vi "Modules global.vi"() -> ()   [LabVIEW 2017]
panel:
  out "Error message":string="Done."
  in  "Use backup file":bool
  in  "Read/Write":bool
  in  "Do Write/Read":bool
  in  "filename":string="24_Apr_2007"
  in  "DAC Break":bool
  in  "DAC Loop":bool
  in  "DAC Update":bool
  in  "All Info":T1(array[cluster])=[[{"Port"=0, "Line"=0, "Description"="Scope Trigger", "Default"=FALSE}, {"Port"=0, "Line"=1, "Description"="Camera trigger (On=High)", "Default"=FALSE}, {"Port"=0, "Line"=2, "Description"="Shim (F/B, U/D) Relay (On = High)", "Default"=TRUE}, {"Port"=0, "Line"=3, "Description"="Shim (L/R) Relay (On = High)", "Default"=TRUE}, {"Port"=0, "Line"=4, "Description"="Rb Trap shutter (High = On)", "Default"=TRUE}, {"Port"=0, "Line"=5, "Description"="", "Default"=FALSE}, {"Port"=0, "Line"=6, "Description"="**//bad TTL//", "Default"=FALSE}, {"Port"=0, "Line"=7, "Description"="Rb F=2 probe shutter", "Default"=FALSE}, {"Port"=0, "Line"=8, "Description"="Rb repump shutter", "Default"=TRUE}, {"Port"=0, "Line"=9, "Description"="Na trap Shutter (On=high)", "Default"=TRUE}, {"Port"=0, "Line"=10, "Description"="Na repump shutter(on)", "Default"=TRUE}, {"Port"=0, "Line"=11, "Description"="optical trap on/off", "Default"=FALSE}, {"Port"=0, "Line"=12, "Description"="Na repump VCO TTL", "Default"=TRUE}, {"Port"=0, "Line"=13, "Description"="Na repump II shtter", "Default"=FALSE}, {"Port"=0, "Line"=14, "Description"="Na trap VCO TTL", "Default"=TRUE}, {"Port"=0, "Line"=15, "Description"="Na F = 2 probe VCO TTL", "Default"=FALSE}], [{"Port"=1, "Line"=0, "Description"="UV LED (On=High)", "Default"=FALSE}, {"Port"=1, "Line"=1, "Description"="Rb F = 2 probe VCO TTL", "Default"=FALSE}, {"Port"=1, "Line"=2, "Description"="", "Default"=FALSE}, {"Port"=1, "Line"=3, "Description"="Track Trigger (Low=MOT)", "Default"=FALSE}, {"Port"=1, "Line"=4, "Description"="Quad enable (High=enabled)", "Default"=FALSE}, {"Port"=1, "Line"=5, "Description"="Bias Multiplexer enable (High=enabled)", "Default"=FALSE}, {"Port"=1, "Line"=6, "Description"="**//bad TTL//", "Default"=FALSE}, {"Port"=1, "Line"=7, "Description"="Rb Repump AOM", "Default"=TRUE}, {"Port"=1, "Line"=8, "Description"="shutter for blocking probe direction", "Default"=FALSE}, {"Port"=1, "Line"=9, "Description"="OP magnetic coil", "Default"=FALSE}, {"Port"=1, "Line"=10, "Description"="\"1\" control bit  for Bias servo mux", "Default"=FALSE}, {"Port"=1, "Line"=11, "Description"="\"2\" control bit  for Bias servo mux", "Default"=FALSE}, {"Port"=1, "Line"=12, "Description"="triggering Agilent frequency sweep for ARPing", "Default"=FALSE}, {"Port"=1, "Line"=13, "Description"="triggering Agilent ramp for frequency sweep", "Default"=FALSE}, {"Port"=1, "Line"=14, "Description"="Na probe shutter", "Default"=FALSE}, {"Port"=1, "Line"=15, "Description"="RF switch for Evap of Rb", "Default"=FALSE}], [{"Port"=2, "Line"=0, "Description"="Feshbach coil switch enable", "Default"=FALSE}, {"Port"=2, "Line"=1, "Description"="Feshbach coil switch polarity", "Default"=FALSE}, {"Port"=2, "Line"=2, "Description"="< line unused>", "Default"=FALSE}, {"Port"=2, "Line"=3, "Description"="690 nm Raman Laser shutter", "Default"=FALSE}, {"Port"=2, "Line"=4, "Description"="< line unused>", "Default"=FALSE}, {"Port"=2, "Line"=5, "Description"="< line unused>", "Default"=FALSE}, {"Port"=2, "Line"=6, "Description"="**//bad TTL//", "Default"=FALSE}, {"Port"=2, "Line"=7, "Description"="< line unused>", "Default"=FALSE}, {"Port"=2, "Line"=8, "Description"="E-field plate switch", "Default"=FALSE}, {"Port"=2, "Line"=9, "Description"=" Ti:sapphire (Raman) shutter", "Default"=FALSE}, {"Port"=2, "Line"=10, "Description"="Raman lasers AOM", "Default"=FALSE}, {"Port"=2, "Line"=11, "Description"="STIRAP waveform trigger", "Default"=FALSE}, {"Port"=2, "Line"=12, "Description"="magic box  RF switch", "Default"=FALSE}, {"Port"=2, "Line"=13, "Description"="Na blast AOM", "Default"=FALSE}, {"Port"=2, "Line"=14, "Description"="< line unused >", "Default"=FALSE}, {"Port"=2, "Line"=15, "Description"="new camera trigger (still connected?)", "Default"=FALSE}], [{"Port"=3, "Line"=0, "Description"="IPG AOM trigger", "Default"=FALSE}, {"Port"=3, "Line"=1, "Description"="660 nm laser (probe) AOM", "Default"=FALSE}, {"Port"=3, "Line"=2, "Description"="< line unused>", "Default"=FALSE}, {"Port"=3, "Line"=3, "Description"="< line unused >", "Default"=FALSE}, {"Port"=3, "Line"=4, "Description"="Pinch servo multiplexer enable", "Default"=FALSE}, {"Port"=3, "Line"=5, "Description"="< line unused >", "Default"=FALSE}, {"Port"=3, "Line"=6, "Description"="**//bad TTL//", "Default"=FALSE}, {"Port"=3, "Line"=7, "Description"="< line unused >", "Default"=FALSE}, {"Port"=3, "Line"=8, "Description"="enable STIRAP back Raman AOM freq shift", "Default"=FALSE}, {"Port"=3, "Line"=9, "Description"="< line unused>", "Default"=FALSE}, {"Port"=3, "Line"=10, "Description"="< line unused>", "Default"=FALSE}, {"Port"=3, "Line"=11, "Description"="< line unused >", "Default"=FALSE}, {"Port"=3, "Line"=12, "Description"="< line unused >", "Default"=FALSE}, {"Port"=3, "Line"=13, "Description"="Dynamic DAC Trigger", "Default"=FALSE}, {"Port"=3, "Line"=14, "Description"="Board 1 Clock Trigger", "Default"=FALSE}, {"Port"=3, "Line"=15, "Description"="Board 2 Clock Trigger", "Default"=FALSE}]]
  in  "File names":string[](array[string])=["MOT recapture", "Most recent expt", "Quadrupole trap", "MOT fill", "BEC", "FORT with transfers", "ZP beam align", "Test1", "Test2", "Align probe beam", "Test3", "Test4", "Test5", "Blank", "Roundtrip MOT recapture", "IP trap load recapture"]
  in  "Modules":string[](array[string])=["Atom removal 1", "Atom removal 2", "B-field off", "CMOT", "Defaults", "Final B-field ramps", "Fluorescence pulse", "High field", "High field ARP", "Loading cart QT", "Loading sci QT", "Low field", "Low field ARP", "Mol OD image", "Mol picture", "Mol probe pulse", "Molasses", "MOT off", "MOT on", "OD image", "Optical pumping", "OT B-field off", "Picture", "Probe pulse", "QT off for OT", "Quadrupole trap off", "Quadrupole trap", "Quantization axis", "S-G separation", "STIRAP back for imaging", "STIRAP", "TTL high", "TTL low", "GPIB", "Utility Module 1", "Utility Module 2", "Utility Module 3", "Utility Module 4", "Utility Module 5", "Utility Module 6", "Utility Module 7", "Utility Module 8", "Utility Module 9"]
  # "0\n\n1\n\n2\n\n3\n\n4\n\n5\n\n6\n\n7\n\n8\n\n9\n\n10\n\n11\n\n12\n\n13\n\n14\n\n15\n\n16\n\n17\n\n18\n\n19\n\n20\n\n21\n\n22\n\n23\n\n24\n\n25\n\n26\n\n27\n\n28\n\n29\n\n30\n\n31\n\n32\n\n33\n\n34\n\n35\n\n36\n\n37\n\n38\n\n39\n\n40\n\n41\n\n42\n\n43\n\n44\n\n45\n\n46\n\n47\n\n48"
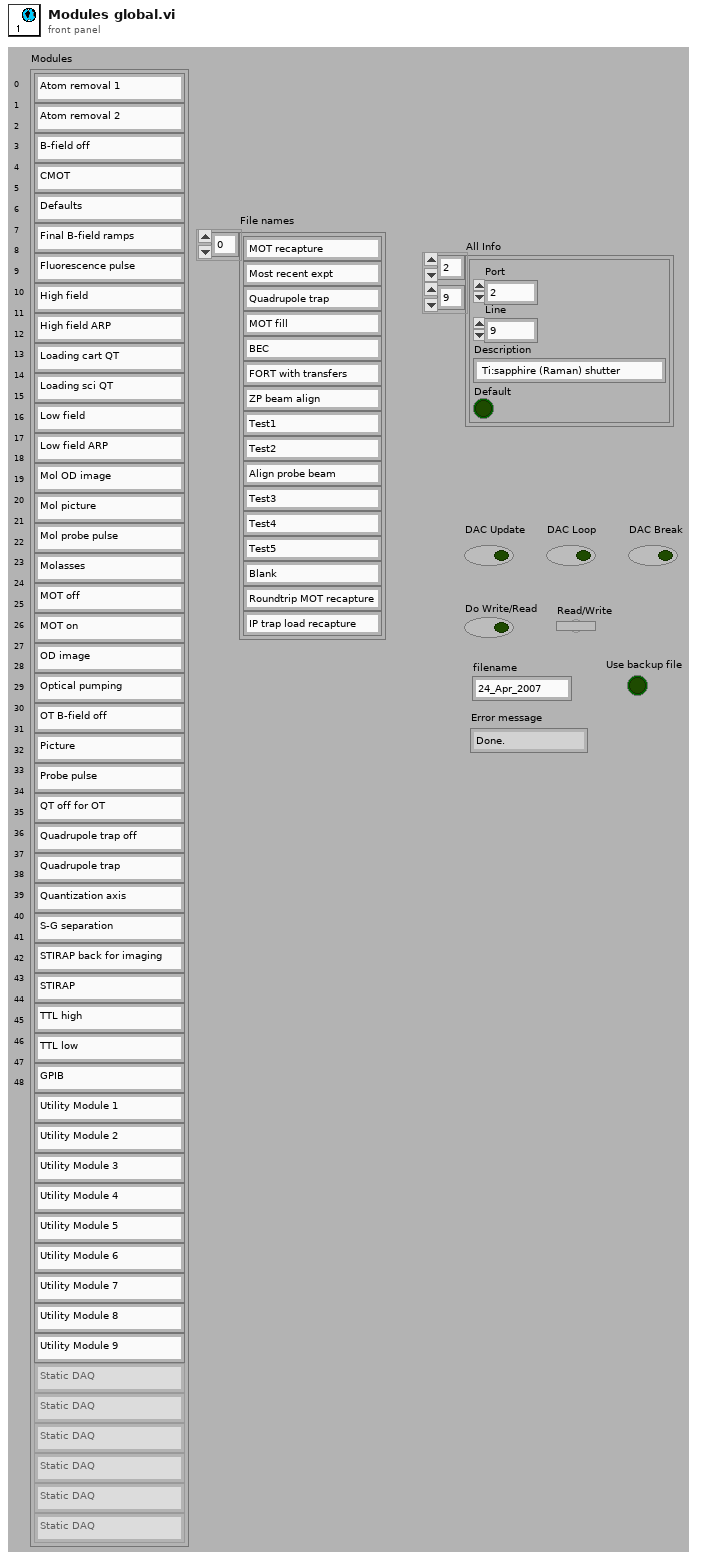
[diagram p1: front panel]
types:
  T1 = cluster{"Port":u32, "Line":u32, "Description":string, "Default":bool}[][]
diagram:
